vi "Read Output Voltage Current.vi"(8 "error in (no error)":errorcluster, 9 "channel (1)":u8=1 min=1 max=4 step=1, 11 "VISA resource name":refnum<visa-resource-name>) -> (0 "error out":errorcluster, 1 "output current":dbl format="%.4f", 2 "output voltage":dbl format="%.4f", 3 "VISA resource name out":refnum<visa-resource-name>)   [LabVIEW 2020, in "Agilent 6XXX Series.lvlib"]
doc: "This function measures the output voltage and current."
uses:
  <instrlib>/Agilent 6XXX Series/Agilent 6XXX Series.lvlib
panel:
  # "*662xA only"
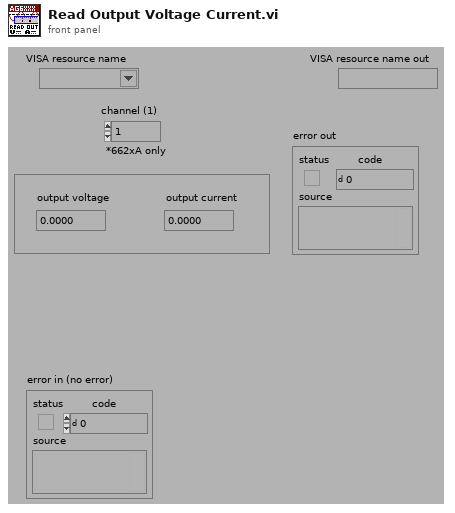
[diagram p1: front panel]
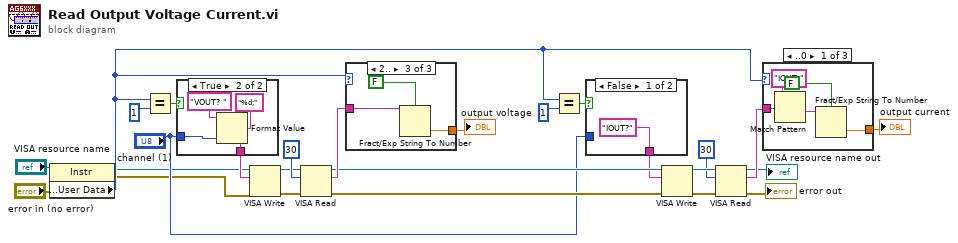
[diagram p0: block diagram]
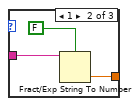
[diagram p2: hidden frame]
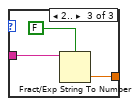
[diagram p3: hidden frame]
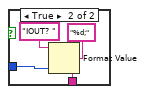
[diagram p4: hidden frame]
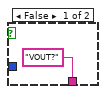
[diagram p5: hidden frame]
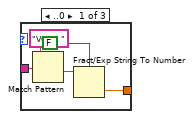
[diagram p6: hidden frame]
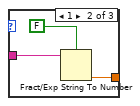
[diagram p7: hidden frame]
diagram:
  n1 = property class="Instr"(reference="VISA resource name", error in="error in (no error)") -> (reference out=w1:refnum<visa-resource-name>, error out=w2:errorcluster, "General Settings:User Data"=w5:u32)
  n2 = Equal?(x=w5, y=u32 1) -> (x = y?=w21:bool)
  n3 = case shown="True" w21 {
    tunnel: ["VOUT?" w28] -> w20
    tunnel: "channel (1)" -> [_ w29]
    frame False {
    }
    frame True {
      n4 = Format Value(string ("")="VOUT? ", format string="%d;", value (0)=w29) -> (output string=w28:string)
    }
  }
  n5 = VISA Write(VISA resource name=w1, write buffer=w20, error in (no error)=w2) -> (VISA resource name out=w25:refnum<visa-resource-name>, error out=w24:errorcluster)  [unwired: 1 out]
  n6 = VISA Read(VISA resource name=w25, byte count=u32 30, error in (no error)=w24) -> (VISA resource name out=w14:refnum<visa-resource-name>, read buffer=w23:string, error out=w15:errorcluster)  [unwired: 1 out]
  n7 = case shown="2.." w5 {
    tunnel: w23 -> [w35 w38 w41]
    tunnel: [w34 w39 w42] -> w19
    frame ..0 {
      n8 = Match Pattern(string=w35, regular expression="VOUT ") -> (after substring=w33:string)  [unwired: 1 in, 3 out]
      n9 = Fract/Exp String To Number(use system decimal point (T)=FALSE, string=w33) -> (number=w34:dbl)  [unwired: 2 in, 1 out]
    }
    frame 1 {
      n10 = Fract/Exp String To Number(use system decimal point (T)=FALSE, string=w38) -> (number=w39:dbl)  [unwired: 2 in, 1 out]
    }
    frame 2.. {
      n11 = Fract/Exp String To Number(use system decimal point (T)=FALSE, string=w41) -> (number=w42:dbl)  [unwired: 2 in, 1 out]
    }
  }
  "output voltage" <- w19
  n12 = Equal?(x=w5, y=u32 1) -> (x = y?=w13:bool)
  n13 = case shown="False" w13 {
    tunnel: ["IOUT?" w44] -> w10
    tunnel: "channel (1)" -> [_ w45]
    frame False {
    }
    frame True {
      n14 = Format Value(string ("")="IOUT? ", format string="%d;", value (0)=w45) -> (output string=w44:string)
    }
  }
  n15 = VISA Write(VISA resource name=w14, write buffer=w10, error in (no error)=w15) -> (VISA resource name out=w17:refnum<visa-resource-name>, error out=w18:errorcluster)  [unwired: 1 out]
  n16 = VISA Read(VISA resource name=w17, byte count=u32 30, error in (no error)=w18) -> (VISA resource name out=→"VISA resource name out":refnum<visa-resource-name>, read buffer=w9:string, error out=→"error out":errorcluster)  [unwired: 1 out]
  n17 = case shown="..0" w5 {
    tunnel: w9 -> [w51 w54 w57]
    tunnel: [w50 w55 w58] -> w6
    frame ..0 {
      n18 = Match Pattern(string=w51, regular expression="IOUT ") -> (after substring=w49:string)  [unwired: 1 in, 3 out]
      n19 = Fract/Exp String To Number(use system decimal point (T)=FALSE, string=w49) -> (number=w50:dbl)  [unwired: 2 in, 1 out]
    }
    frame 1 {
      n20 = Fract/Exp String To Number(use system decimal point (T)=FALSE, string=w54) -> (number=w55:dbl)  [unwired: 2 in, 1 out]
    }
    frame 2.. {
      n21 = Fract/Exp String To Number(use system decimal point (T)=FALSE, string=w57) -> (number=w58:dbl)  [unwired: 2 in, 1 out]
    }
  }
  "output current" <- w6
